vi "Calculate Clock Settings.vi"(4 "Coerce Range?":bool, 5 "Max Frequency (Hz)":dbl, 6 "Phase Correct Mode?":bool, 7 "Min Frequency (Hz)":dbl, 8 "error in (no error)":errorcluster, 9 "Requested Frequency (Hz)":dbl, 10 "Clock Calculation Parameters":T1={"Base Clock Frequency (Hz)"=40000000.0, "Max Counter Value"=65535, "Min Counter Value"=100}, 11 "Clock Divisors":u32[](array[numeric])=[1, 2, 4, 8, 16]) -> (0 "error out":errorcluster, 3 "Frequency Configuration":T2 {"Actual Frequency (Hz)" format="%#.2f"})   [LabVIEW 2021]
uses:
  <vilib>/myRIO/Common/Instrument Driver Framework/Utilities/typedefs/Clock Settings.ctl
  <vilib>/myRIO/Common/Instrument Driver Framework/Utilities/typedefs/Clock Calculation Parameters.ctl
panel:
  # "NOTE:\nThe Requested Frequency input needs to be greater than 0 for this VI to work correctly."
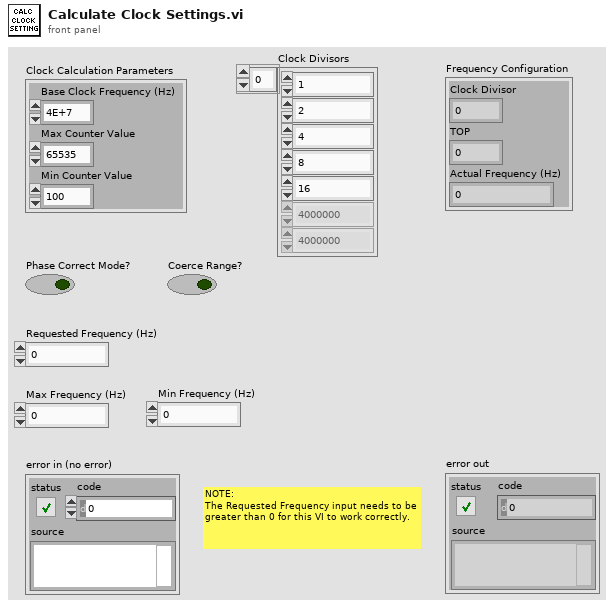
[diagram p1: front panel]
types:
  T1 = typedef "Clock Calculation Parameters.ctl" = cluster{"Base Clock Frequency (Hz)":dbl, "Max Counter Value":u32, "Min Counter Value":u32}
  T2 = typedef "Clock Settings.ctl" = cluster{"Clock Divisor":u32, "TOP":u32, "Actual Frequency (Hz)":dbl}
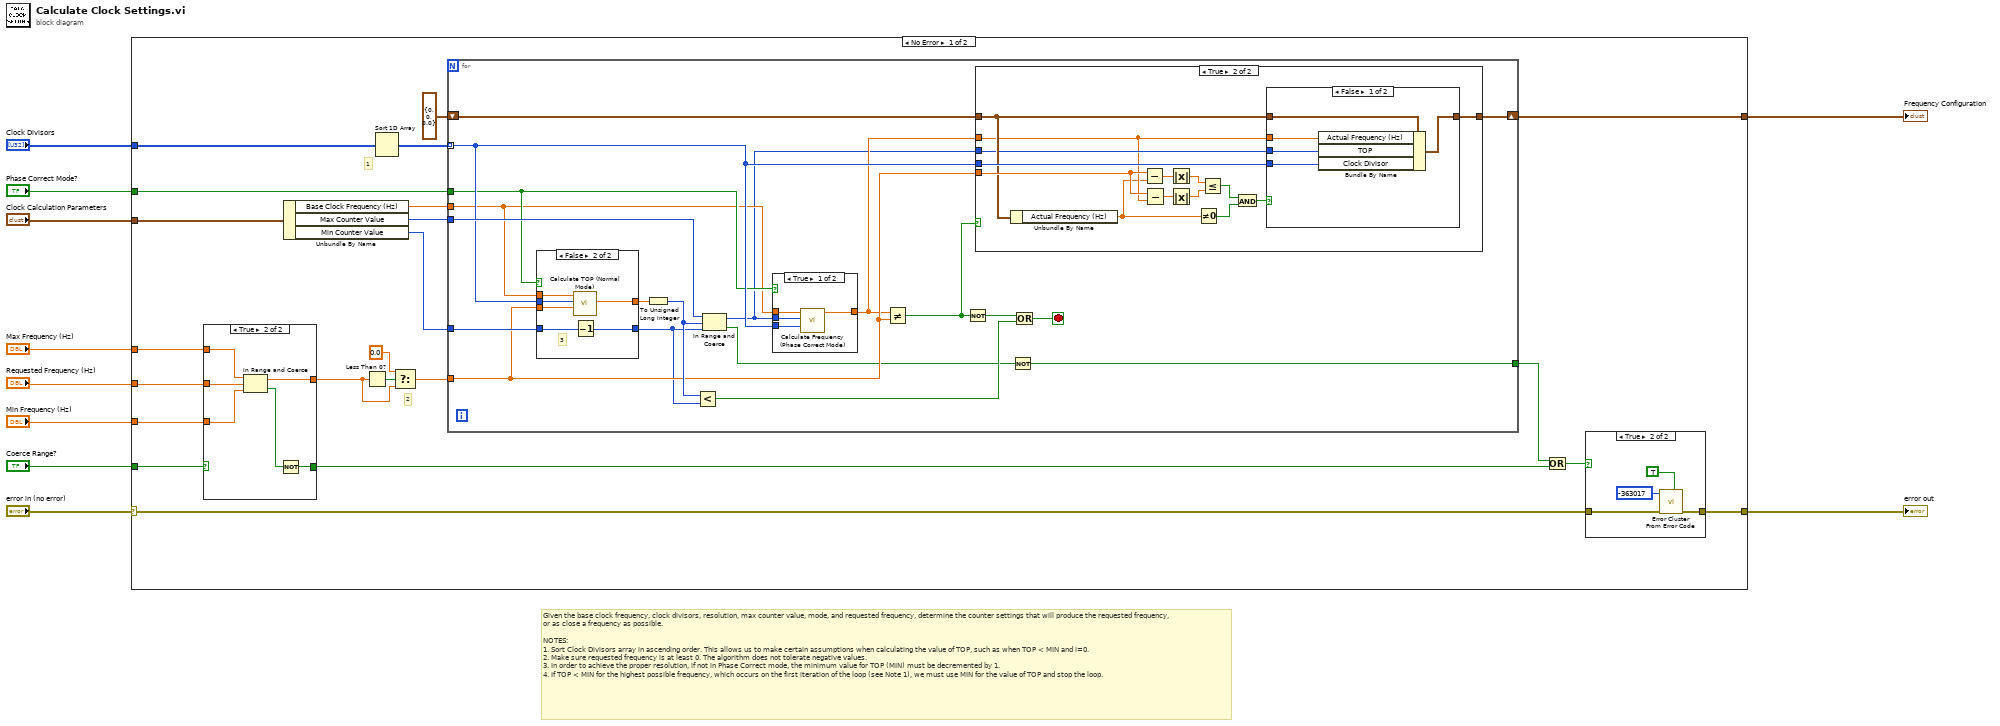
[diagram p0: block diagram]
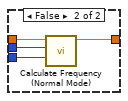
[diagram p3: hidden frame]
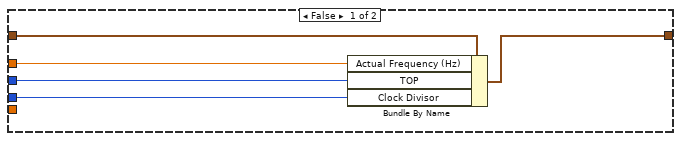
[diagram p4: hidden frame]
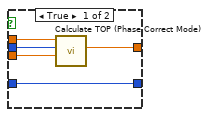
[diagram p6: hidden frame]
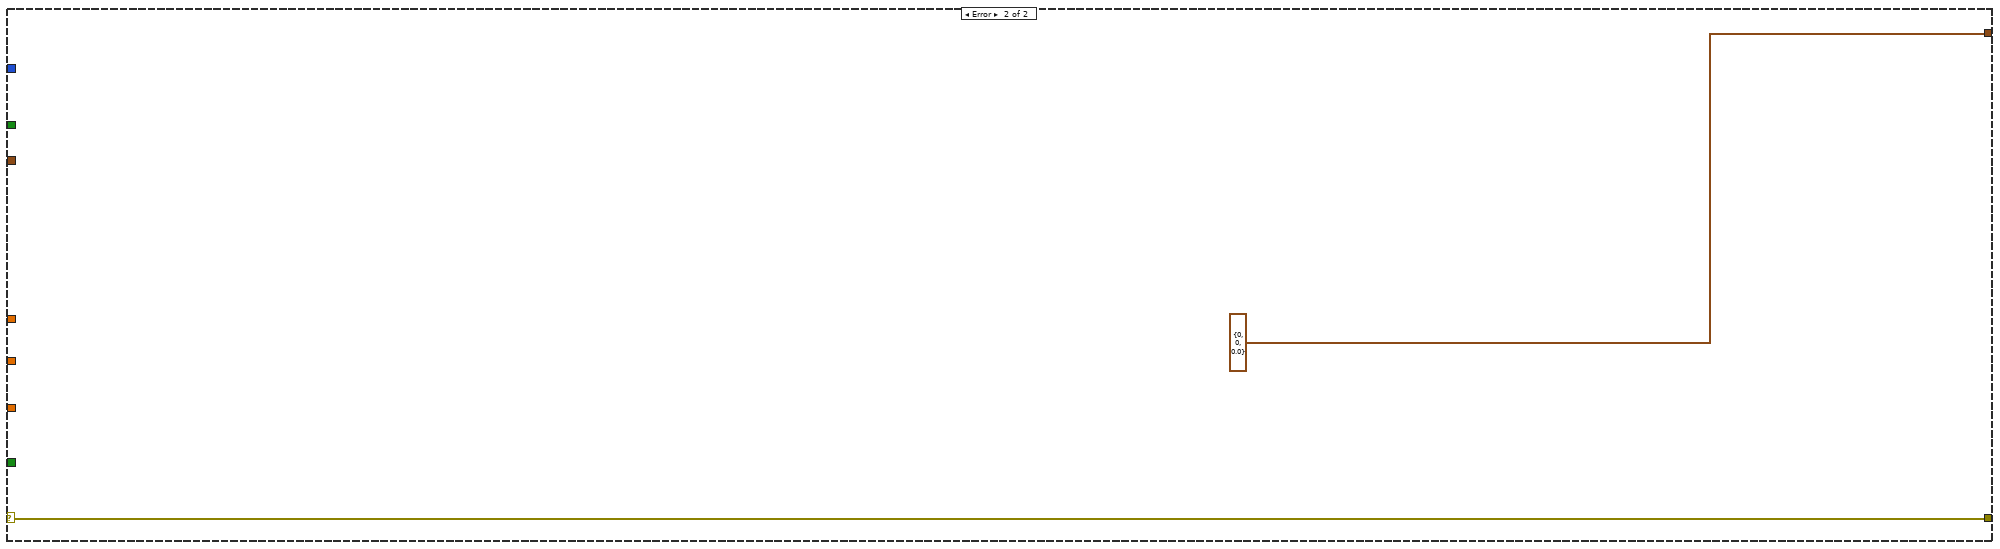
[diagram p8: hidden frame]
diagram:
  # "Given the base clock frequency, clock divisors, resolution, max counter value, mode, and requested frequency, determine the counter settings that will produce the requested frequency, or as close a frequency as possible.\n\nNOTES:\n1. Sort Clock Divisors array in ascending order. This allows us to make certain assumptions when calculating the value of TOP, such as when TOP < MIN and i=0.\n2. Make sure requested frequency is at least 0. The algorithm does not tolerate negative values.\n3. In order to achieve the proper resolution, if not in Phase Correct mode, the minimum value for TOP (MIN) must be decremented by 1.\n4. If TOP < MIN for the highest possible frequency, which occurs on the first iteration of the loop (see Note 1), we must use MIN for the value of TOP and stop the loop."
  n1 = case shown="No Error" "error in (no error)" {
    selector: "error in (no error)" -> [w13 w110]
    tunnel: "Clock Divisors" -> [w32 _]
    tunnel: "Phase Correct Mode?" -> [w30 _]
    tunnel: [w28 T2 {"Clock Divisor"=0, "TOP"=0, "Actual Frequency (Hz)"=0.0} ("Frequency Configuration")] -> w8
    tunnel: "Clock Calculation Parameters" -> [w12 _]
    tunnel: [w24 w110] -> w6
    tunnel: "Max Frequency (Hz)" -> [w20 _]
    tunnel: "Min Frequency (Hz)" -> [w19 _]
    tunnel: "Requested Frequency (Hz)" -> [w18 _]
    tunnel: "Coerce Range?" -> [w17 _]
    frame No Error {
      # "2"
      # "1"
      n2 = case shown="True" w17 {
        selector: w17 -> [w33 _]
        tunnel: w20 -> [_ w40]
        tunnel: w19 -> [_ w39]
        tunnel: w18 -> [w34 w38]
        tunnel: [w34 w37] -> w16
        tunnel: [w33 w35] -> w14
        frame False {
        }
        frame True {
          n3 = In Range and Coerce(upper limit=w40, x=w38, lower limit=w39) -> (coerced(x)=w37:dbl, In Range?=w36:bool)
          n4 = Not(x=w36) -> (.not. x?=w35:bool)
        }
      }
      n5 = Unbundle By Name(w12) -> ("Base Clock Frequency (Hz)"=w27:dbl, "Max Counter Value"=w26:u32, "Min Counter Value"=w25:u32)
      n6 = Less Than 0?(x=w16) -> (x < 0?=w22:bool)
      n7 = Sort 1D Array(array=w32) -> (sorted array=w31:u32[])
      n8 = Select(t=0.0, s=w22, f=w16) -> (s? t:f=w23:dbl)
      n9 = for {
        tunnel: w31 -> [w52] mode=indexing
        tunnel: w30 -> [w50]
        tunnel: w26 -> [w56]
        tunnel: w25 -> [w53]
        shift-right: [w57] -> w28
        shift-left: T2 {"Clock Divisor"=0, "TOP"=0, "Actual Frequency (Hz)"=0.0} ("Frequency Configuration") -> [w58]
        tunnel: w27 -> [w48]
        tunnel: w23 -> [w49]
        tunnel: [w42] -> w11
        stop <- w59 stop-if-true
        n10 = case shown="False" w50 {
          tunnel: w48 -> [w97 w103]
          tunnel: [w96 w102] -> w55
          tunnel: w52 -> [w95 w101]
          tunnel: w53 -> [w94 w100]
          tunnel: [w94 w99] -> w41
          tunnel: w49 -> [w93 w98]
          frame True {
            n11 = call <vilib>:"Calculate TOP (Phase Correct Mode).vi"("Requested Frequency (Hz)"=w93, "Clock Divisor"=w95, "Base Clock Frequency (Hz)"=w97) -> ("TOP"=w96:dbl)  [unwired: 7 in, 1 out]
          }
          frame False {
            # "3"
            n12 = call <vilib>:"Calculate TOP (Normal Mode).vi"("Requested Frequency (Hz)"=w98, "Clock Divisor"=w101, "Base Clock Frequency (Hz)"=w103) -> ("TOP"=w102:dbl)  [unwired: 7 in, 1 out]
            n13 = Decrement(x=w100) -> (x-1=w99:u32)
          }
        }
        n14 = To Unsigned Long Integer(number=w55) -> (unsigned 32bit integer=w54:u32)
        n15 = Less?(x=w54, y=w41) -> (x < y?=w51:bool)
        n16 = In Range and Coerce(upper limit=w56, x=w54, lower limit=w41) -> (coerced(x)=w44:u32, In Range?=w43:bool)
        n17 = case shown="True" w50 {
          tunnel: [w63 w67] -> w45
          tunnel: w48 -> [w62 w66]
          tunnel: w44 -> [w61 w64]
          tunnel: w52 -> [w60 w65]
          frame True {
            n18 = call <vilib>:"Calculate Frequency (Phase Correct Mode).vi"("Clock Divisor"=w60, "TOP"=w61, "Base Clock Frequency (Hz)"=w62) -> ("Frequency (Hz)"=w63:dbl)  [unwired: 8 in]
          }
          frame False {
            n19 = call <vilib>:"Calculate Frequency (Normal Mode).vi"("Clock Divisor"=w65, "TOP"=w64, "Base Clock Frequency (Hz)"=w66) -> ("Frequency (Hz)"=w67:dbl)  [unwired: 8 in]
          }
        }
        n20 = Not Equal?(x=w45, y=w49) -> (x != y?=w46:bool)
        n21 = Not(x=w46) -> (.not. x?=w47:bool)
        n22 = case shown="True" w46 {
          tunnel: w58 -> [w72 w80]
          tunnel: w52 -> [w70 w86]
          tunnel: w49 -> [_ w81]
          tunnel: [w71 w79] -> w57
          tunnel: w45 -> [w69 w77]
          tunnel: w44 -> [w68 w78]
          frame False {
            n23 = Bundle By Name(cluster=w72, "Actual Frequency (Hz)"=w69, "TOP"=w68, "Clock Divisor"=w70) -> (w71:T2)
          }
          frame True {
            n24 = Unbundle By Name(w80) -> ("Actual Frequency (Hz)"=w76:dbl)
            n25 = Subtract(x=w81, y=w76) -> (x-y=w85:dbl)
            n26 = Subtract(x=w81, y=w77) -> (x-y=w83:dbl)
            n27 = Absolute Value(x=w85) -> (abs(x)=w84:dbl)
            n28 = Absolute Value(x=w83) -> (abs(x)=w82:dbl)
            n29 = Not Equal To 0?(x=w76) -> (x != 0?=w74:bool)
            n30 = Less Or Equal?(x=w84, y=w82) -> (x <= y?=w73:bool)
            n31 = And(x=w73, y=w74) -> (x .and. y?=w75:bool)
            n32 = case shown="False" w75 {
              tunnel: w86 -> [w89 _]
              tunnel: w80 -> [w91 w92]
              tunnel: [w90 w92] -> w79
              tunnel: w77 -> [w88 _]
              tunnel: w78 -> [w87 _]
              frame False {
                n33 = Bundle By Name(cluster=w91, "Actual Frequency (Hz)"=w88, "TOP"=w87, "Clock Divisor"=w89) -> (w90:T2)
              }
              frame True {
              }
            }
          }
        }
        n34 = Not(x=w43) -> (.not. x?=w42:bool)
        n35 = Or(x=w47, y=w51) -> (x .or. y?=w59:bool)
      }
      n36 = Or(x=w11, y=w14) -> (x .or. y?=w15:bool)
      n37 = case shown="True" w15 {
        tunnel: w13 -> [w104 w108]
        tunnel: [w104 w107] -> w24
        frame False {
        }
        frame True {
          n38 = call <vilib>:"Error Cluster From Error Code.vi"("is warning? (False)"=TRUE, "error in (no error)"=w108, "error code (0)"=-363017) -> ("error out"=w107:errorcluster)  [unwired: 6 in]
        }
      }
    }
    frame Error {
    }
  }
  "Frequency Configuration" <- w8
  "error out" <- w6
